vi "FPGA TimeTag.vi"(7 "runs":i32, 8 "error in (no error)":errorcluster, 9 "fileName":string, 10 "fpgaCommand":u8, 11 "saveData":bool) -> (0 "error out":errorcluster, 3 "function return":i32, 4 "stats":i64[](array[numeric]))   [LabVIEW 2015]
uses:
  x64/Stats.lvlib
  x86/Stats32.lvlib
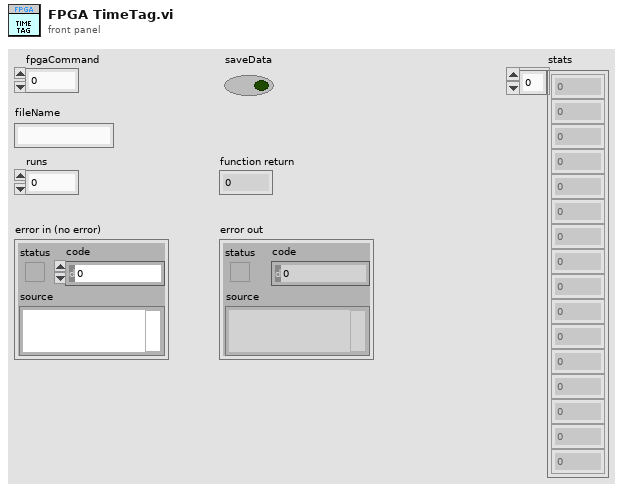
[diagram p1: front panel]
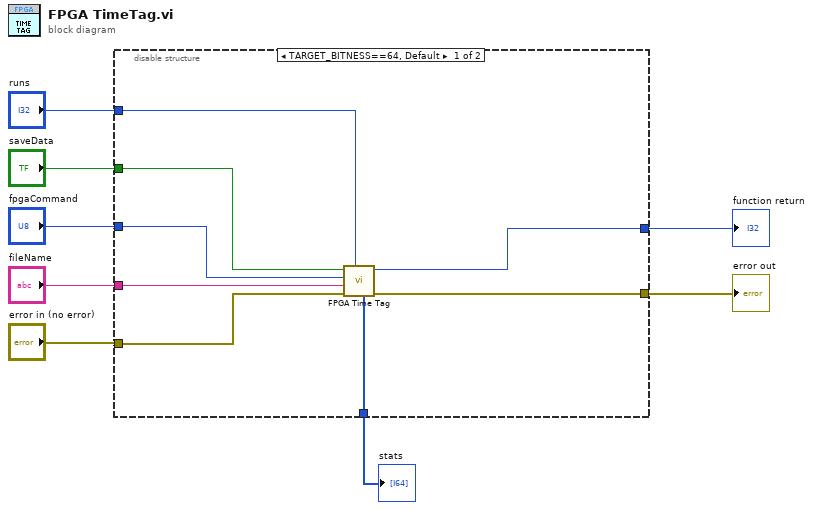
[diagram p0: block diagram]
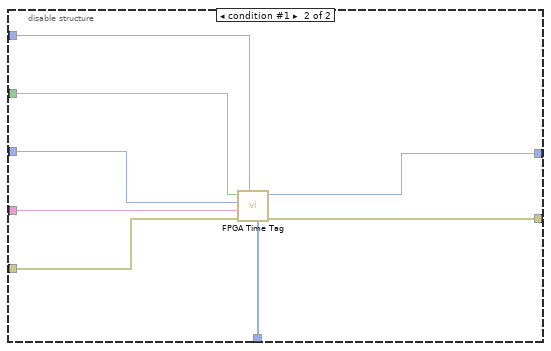
[diagram p2: hidden frame]
diagram:
  n1 = disable-structure shown="TARGET_BITNESS==64, Default" {
    disable-tunnel: "error in (no error)" -> [w16 w22]
    disable-tunnel: [w15 w24] -> w7
    disable-tunnel: [w14 w23] -> w6
    disable-tunnel: "saveData" -> [w13 w19]
    disable-tunnel: "fpgaCommand" -> [w12 w20]
    disable-tunnel: "fileName" -> [w11 w21]
    disable-tunnel: "runs" -> [w10 w18]
    disable-tunnel: [w9 w17] -> w1
    frame condition #0 (active) {
      n2 = call "FPGA Time Tag.vi"("runs"=w10, "error in (no error)"=w16, "fileName"=w11, "fpgaCommand"=w12, "saveClicks"=w13) -> ("error out"=w15:errorcluster, "function return"=w14:i32, "stats"=w9:i64[])  [unwired: 3 in, 1 out]
    }
    frame condition #1 {
      n3 = call "FPGA Time Tag.vi"("runs"=w18, "error in (no error)"=w22, "fileName"=w21, "fpgaCommand"=w20, "saveClicks"=w19) -> ("error out"=w24:errorcluster, "function return"=w23:i32, "Stats"=w17:i32[])  [unwired: 4 in]
    }
  }
  "error out" <- w7
  "function return" <- w6
  "stats" <- w1
